vi "Sql.vi"() -> ()   [LabVIEW 2024]
uses:
  <vilib>/drjdpowell/SQLite Library/SQL Connection/Open (path).vi
  <vilib>/drjdpowell/SQLite Library/SQL Connection/Open (string).vi
  <vilib>/AdvancedString/Path To Command Line String.vi
  <vilib>/drjdpowell/SQLite Library/SQL Connection/Execute SQL (Single String).vi
  <vilib>/drjdpowell/SQLite Library/SQL Connection/Connection.lvclass
  <vilib>/drjdpowell/SQLite Library/SQLite.lvlib
panel:
  in  "基路径":path
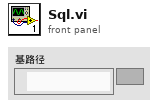
[diagram p1: front panel]
types:
  T1 = enum16{"New or existing", "Existing", "Read only"}
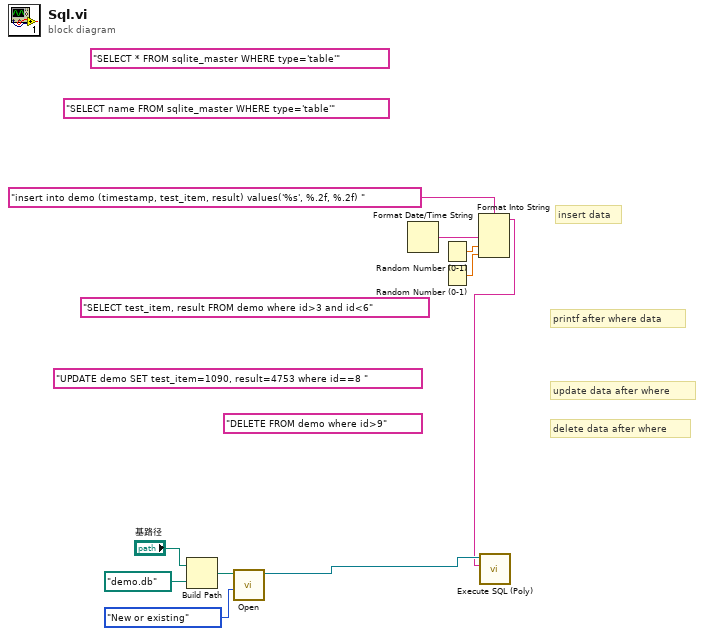
[diagram p0: block diagram]
diagram:
  (unwired) "DELETE FROM demo where id>9" ("SQL")
  (unwired) "UPDATE demo SET test_item=1090, result=4753 where id==8 " ("SQL")
  (unwired) "SELECT test_item, result FROM demo where id>3 and id<6" ("SQL")
  (unwired) "SELECT name FROM sqlite_master WHERE type='table'" ("SQL")
  (unwired) "SELECT * FROM sqlite_master WHERE type='table'" ("SQL")
  # "delete data after where"
  # "update data after where"
  # "printf after where data"
  # "insert data"
  n1 = Build Path(base path="基路径", name or relative path=path "demo.db" ("名称或相对路径")) -> (appended path=w4:path)
  n2 = call-poly <vilib>:"Open.vi"("File Option"=T1."New or existing", "db file"=w4) -> ("SQLite Connection"=w2:refnum<class "Connection.lvclass">)  [unwired: 8 in, 1 out]
  n3 = Format Date/Time String() -> (date/time string=w10:string)  [unwired: 3 in]
  n4 = Random Number (0-1)() -> (number: 0 to 1=w8:dbl)
  n5 = Random Number (0-1)() -> (number: 0 to 1=w7:dbl)
  n6 = Format Into String(format string="insert into demo (timestamp, test_item, result) values('%s', %.2f, %.2f) " ("SQL"), w10, w8, w7) -> (resulting string=w1:string)  [unwired: 2 in, 1 out]
  n7 = call-poly <vilib>:"Execute SQL (Poly).vi"("SQL"=w1, "SQLite Connection in"=w2) -> ()  [unwired: 7 in, 3 out]
